vi "mouse_ctrl upd_mark_plot.vi"(8 "error in (no error)":errorcluster, 11 "mouse_ctrl in":refnum<class "mouse_ctrl.lvclass">) -> (0 "error out":errorcluster, 3 "mouse_ctrl out":refnum<class "mouse_ctrl.lvclass">)   [LabVIEW 2018, in "mouse_ctrl.lvclass"]
uses:
  mouse_ctrl.lvclass
  mouse_ctrl.lvclass/mouse_ctrl.ctl
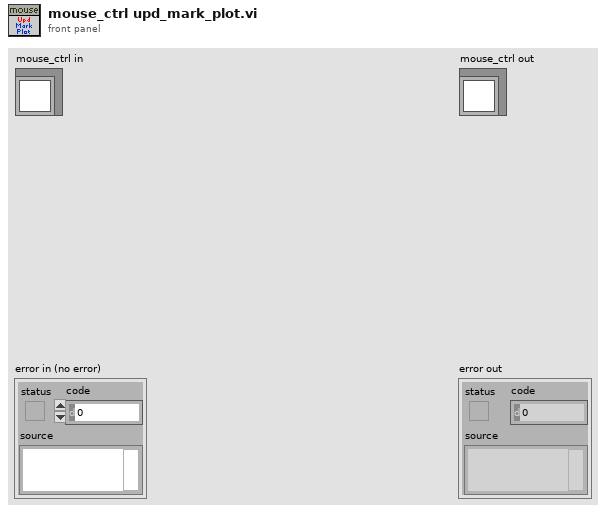
[diagram p1: front panel]
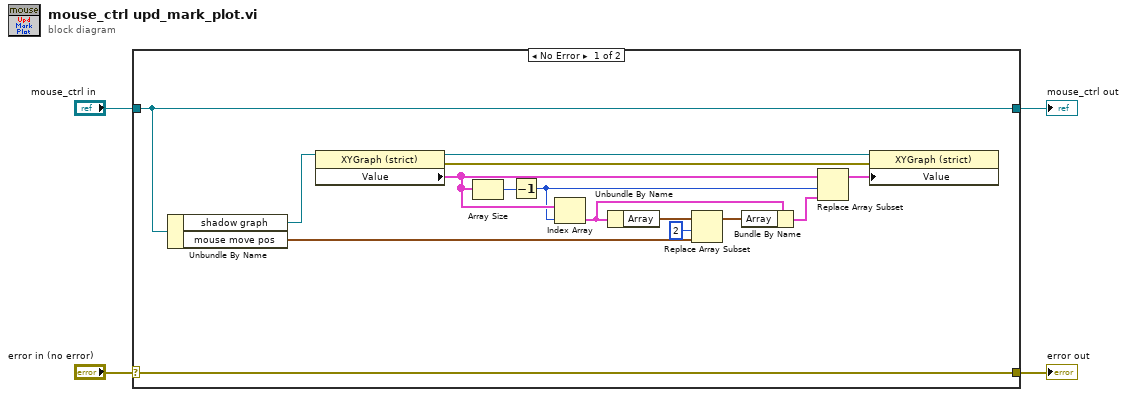
[diagram p0: block diagram]
diagram:
  n1 = case shown="No Error" "error in (no error)" {
    selector: "error in (no error)" -> [w19 w21]
    tunnel: [w19 w21] -> w3
    tunnel: [w18 w20] -> w1
    tunnel: "mouse_ctrl in" -> [w18 w20]
    frame No Error {
      n2 = Unbundle By Name(w18) -> ("shadow graph"=w17:refnum<vi>, "mouse move pos"=w8:cluster{"X":dbl, "Y":dbl})
      n3 = property class="XYGraph (strict)"(reference=w17) -> (reference out=w13:refnum<vi>, error out=w12:errorcluster, "Value"=w15:cluster{"Array":cluster{"X":dbl, "Y":dbl}[]}[])  [unwired: 1 in]
      n4 = Array Size(array=w15) -> (size(s)=w16:i32)
      n5 = Decrement(x=w16) -> (x-1=w14:i32)
      n6 = Index Array(array=w15, index=w14) -> (element=w7:cluster{"Array":cluster{"X":dbl, "Y":dbl}[]})
      n7 = Unbundle By Name(w7) -> ("Array"=w10:cluster{"X":dbl, "Y":dbl}[])
      n8 = Replace Array Subset(array=w10, new element=w8, index=2) -> (w6:cluster{"X":dbl, "Y":dbl}[])
      n9 = Bundle By Name(cluster=w7, "Array"=w6) -> (w5:cluster{"Array":cluster{"X":dbl, "Y":dbl}[]})
      n10 = Replace Array Subset(array=w15, new element=w5, index=w14) -> (w11:cluster{"Array":cluster{"X":dbl, "Y":dbl}[]}[])
      n11 = property class="XYGraph (strict)"(reference=w13, error in=w12, "Value"=w11) -> ()  [unwired: 2 out]
    }
    frame Error {
    }
  }
  "error out" <- w3
  "mouse_ctrl out" <- w1
